vi "thorlabs_zero_piezos.vi"(8 "error in (no error)":errorcluster, 11 "thorlabs_panel in":refnum<class "thorlabs_panel.lvclass">) -> (0 "error out":errorcluster, 3 "thorlabs_panel out":refnum<class "thorlabs_panel.lvclass">)   [LabVIEW 2015, in "thorlabs_panel.lvclass"]
uses:
  thorlabs_panel.lvclass
  thorlabs_class/thorlabs_kinesis.lvclass
  UI/panel_class/panel.lvclass
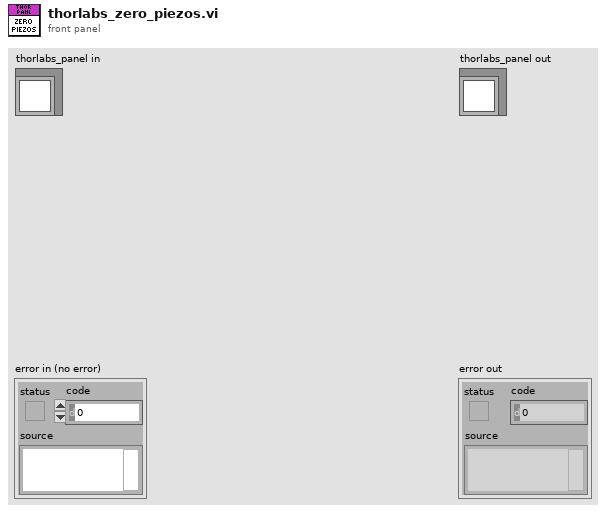
[diagram p1: front panel]
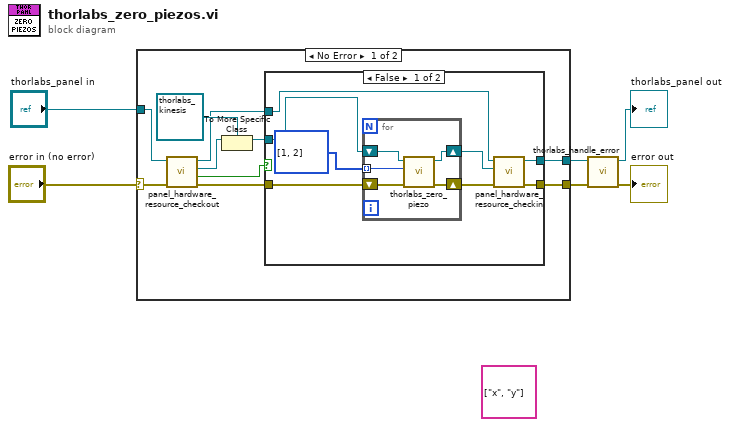
[diagram p0: block diagram]
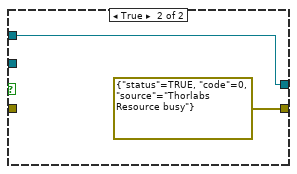
[diagram p2: hidden frame]
diagram:
  (unwired) string[] ["x", "y"]
  n1 = case shown="No Error" "error in (no error)" {
    selector: "error in (no error)" -> [w15 w33]
    tunnel: [w8 w33] -> w1
    tunnel: [w7 w32] -> w4
    tunnel: "thorlabs_panel in" -> [w16 w32]
    frame No Error {
      n2 = call "panel_hardware_resource_checkout.vi"("error in (no error)"=w15, "panel in"=w16) -> ("error out"=w11:errorcluster, "timed out?"=w10:bool, "hardware.lvclass"=w14:refnum<class "hardware.lvclass">, "panel out"=w9:refnum<class "thorlabs_panel.lvclass">)  [unwired: 6 in]
      n3 = To More Specific Class(target class=refnum<class "thorlabs_kinesis.lvclass"> refnum ("thorlabs_kinesis.lvclass"), reference=w14) -> (specific class reference=w12:refnum<class "thorlabs_kinesis.lvclass">)  [unwired: 1 in, 1 out]
      n4 = case shown="False" w10 {
        tunnel: w12 -> [w20 _]
        tunnel: w11 -> [w21 _]
        tunnel: w9 -> [w22 w30]
        tunnel: [w24 w30] -> w7
        tunnel: [w23 errorcluster {"status"=TRUE, "code"=0, "source"="Thorlabs Resource busy"} ("error out")] -> w8
        frame False {
          n5 = for {
            shift-right: [w27] -> w19
            shift-left: w21 -> [w26]
            shift-right: [w28] -> w18
            shift-left: w20 -> [w29]
            tunnel: i32[] [1, 2] -> [w25] mode=indexing
            n6 = call "thorlabs_zero_piezo.vi"("error in (no error)"=w26, "channel"=w25, "thorlabs_kinesis in"=w29) -> ("error out"=w27:errorcluster, "thorlabs_kinesis out"=w28:refnum<class "thorlabs_kinesis.lvclass">)  [unwired: 7 in]
          }
          n7 = call "panel_hardware_resource_checkin.vi"("error in (no error)"=w19, "hardware.lvclass"=w18, "panel in"=w22) -> ("error out"=w23:errorcluster, "panel out"=w24:refnum<class "thorlabs_panel.lvclass">)  [unwired: 7 in]
        }
        frame True {
        }
      }
    }
    frame Error {
    }
  }
  n8 = call "thorlabs_handle_error.vi"("error in (no error)"=w1, "thorlabs_panel in"=w4) -> ("error out"=→"error out":errorcluster, "thorlabs_panel out"=→"thorlabs_panel out":refnum<class "thorlabs_panel.lvclass">)  [unwired: 8 in]
